vi "TCPSend (SubVI).vi"(7 "Opcode":u32=4096 format="%.0x", 8 "error in":errorcluster, 9 "string":string, 10 "Drv":u8, 11 "connection ID":refnum<k5>) -> (0 "error out":errorcluster)   [LabVIEW 2017]
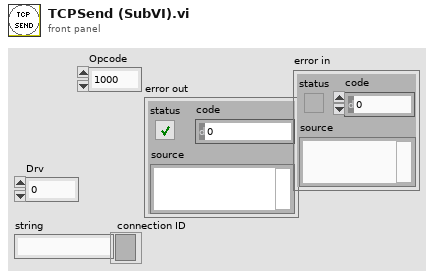
[diagram p1: front panel]
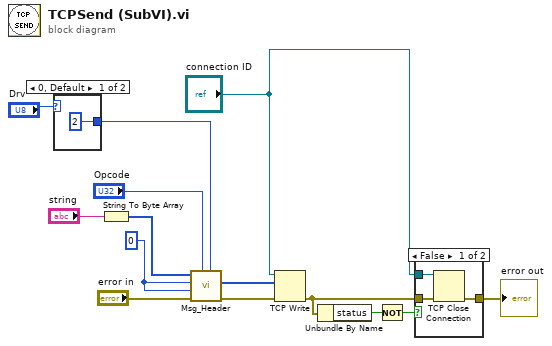
[diagram p0: block diagram]
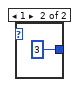
[diagram p2: hidden frame]
diagram:
  w8 = u32 0 ("Source")
  n1 = case shown="0, Default" "Drv" {
    tunnel: [u8 2 u8 3] -> w7
    frame 0, Default {
    }
    frame 1 {
    }
  }
  n2 = String To Byte Array(string="string") -> (unsigned byte array=w9:u8[])
  n3 = call "Msg_Header.vi"("Res1"=w7, "Opcode"="Opcode", "error in"="error in", "Destination"=w8, "Source"=w8, "Dody"=w9) -> ("error out"=w11:errorcluster, "output array"=w10:u8[])  [unwired: 4 in]
  n4 = TCP Write(connection ID="connection ID", data in=w10, error in (no error)=w11) -> (error out=w13:errorcluster)  [unwired: 1 in, 2 out]
  n5 = Unbundle By Name(w13) -> ("status"=w3:bool)
  n6 = Not(x=w3) -> (.not. x?=w4:bool)
  n7 = case shown="False" w4 {
    tunnel: "connection ID" -> [w19 _]
    tunnel: [w18 w20] -> w14
    tunnel: w13 -> [w17 w20]
    frame False {
      n8 = TCP Close Connection(connection ID=w19, error in (no error)=w17) -> (error out=w18:errorcluster)  [unwired: 1 in, 1 out]
    }
    frame True {
    }
  }
  "error out" <- w14
